vi "Set RIO INI Key.vi"(8 "error in (no error)":errorcluster) -> (0 "error out":errorcluster)   [LabVIEW 2016, in "FPGA Addon Engine.lvlib"]
uses:
  FPGA Addon Engine.lvlib
  <vilib>/Utility/config.llb/Write Key (I32).vi
  <vilib>/Utility/config.llb/NI_LVConfig.lvlib
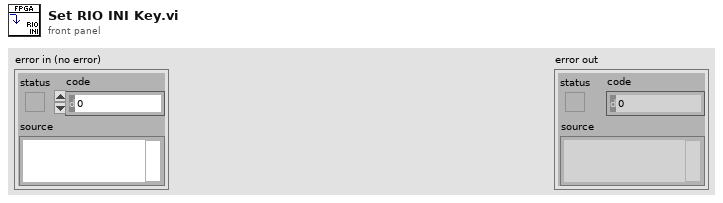
[diagram p1: front panel]
types:
  T1 = typedef "NI_LVConfig.lvlib/Config Data RefNum.ctl" = refnum<k1>
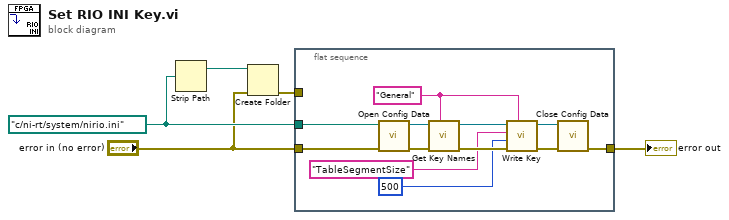
[diagram p0: block diagram]
diagram:
  w4 = path "c:/ni-rt/system/nirio.ini" ("configuration file path")
  n1 = Strip Path(path=w4) -> (stripped path=w3:path)  [unwired: 1 out]
  n2 = Create Folder(path (use dialog)=w3, error in="error in (no error)") -> (error out=w1:errorcluster)  [unwired: 1 in, 2 out]
  n3 = flat-sequence {
    tunnel: [w8] -> w5
    tunnel: w4 -> [w7]
    tunnel: "error in (no error)" -> [w6]
    tunnel: w1 -> [_]
    frame #0 {
      w14 = "General" ("section")
      n4 = call <vilib>:"Open Config Data.vi"("error in (no error)"=w6, "configuration file path"=w7) -> ("error out"=w17:errorcluster, "refnum"=w16:T1)  [unwired: 7 in, 1 out]
      n5 = call <vilib>:"Get Key Names.vi"("section"=w14, "error in (no error)"=w17, "refnum"=w16) -> ("error out"=w13:errorcluster, "refnum out"=w15:T1)  [unwired: 5 in, 2 out]
      n6 = call-poly <vilib>:"Write Key.vi"("section"=w14, "error in (no error)"=w13, "value"=500, "key"="TableSegmentSize", "refnum"=w15) -> ("error out"=w9:errorcluster, "refnum out"=w12:T1)  [unwired: 4 in, 1 out]
      n7 = call <vilib>:"Close Config Data.vi"("error in (no error)"=w9, "refnum"=w12) -> ("error out"=w8:errorcluster)  [unwired: 8 in, 1 out]
    }
  }
  "error out" <- w5
